vi "StaticTextIndicatorstoSaveSpaceonBlockdiogram_171213.vi"() -> (3 "8":string, 4 "KeyboardShortcuts":string, 5 "KejyboardShortcuts2":string, 6 "Statistics":string, 7 "FilterType":string, 8 "CageSegments":string, 9 "TimeSpentinEachSegment":string, 10 "CageSegmentation":string, 11 "AssignedSegments":string, 12 "Border":string, 13 "Center":string, 14 "CurrentDistanceTraveled":string, 15 "DisplayOptions":string, 16 "3":string, 17 "4":string, 18 "ElapsedTimePlayback":string, 19 "12":string, 20 "13":string, 21 "TIme1":string, 22 "11":string, 23 "Time2":string, 24 "10":string, 25 "ElapsedTimeRecording":string, 26 "5":string)   [LabVIEW 2016]
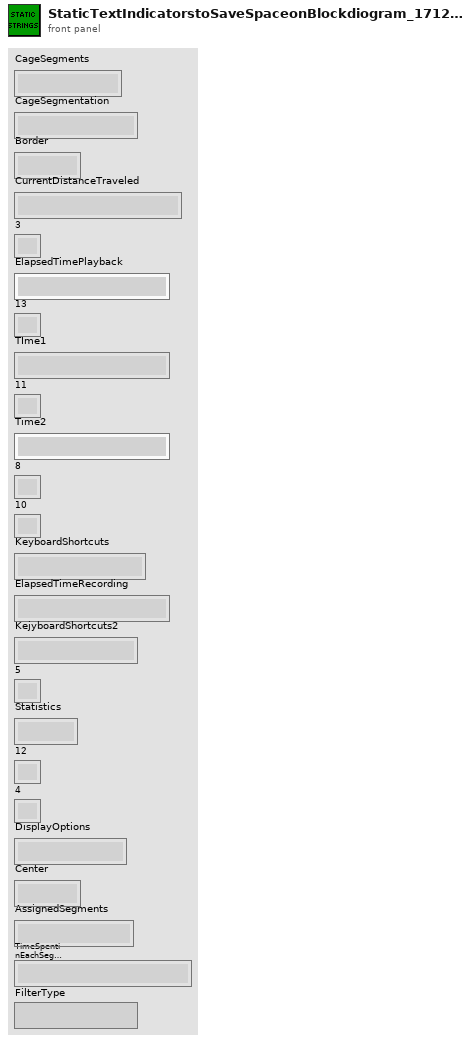
[diagram p1: front panel]
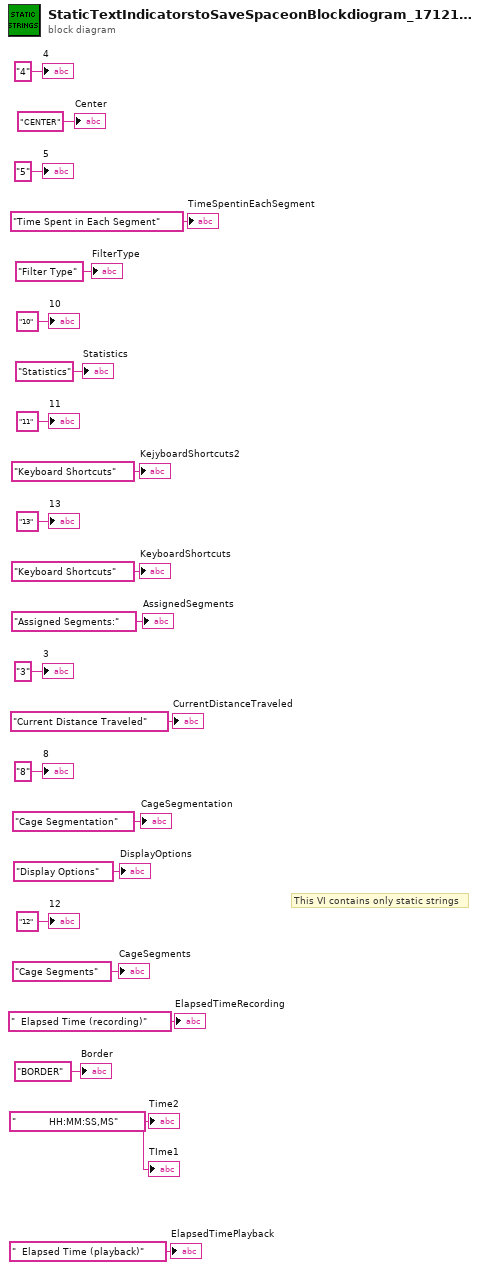
[diagram p0: block diagram]
diagram:
  w6 = "           HH:MM:SS,MS" ("String 5")
  # "This VI contains only static strings"
  "KeyboardShortcuts" <- "Keyboard Shortcuts" ("String 9")
  "Statistics" <- "Statistics" ("String 39")
  "TimeSpentinEachSegment" <- "Time Spent in Each Segment" ("String 40")
  "AssignedSegments" <- "Assigned Segments:" ("String 4")
  "DisplayOptions" <- "Display Options" ("String 35")
  "ElapsedTimeRecording" <- "  Elapsed Time (recording)" ("String")
  "TIme1" <- w6
  "ElapsedTimePlayback" <- "  Elapsed Time (playback)" ("String")
  "Time2" <- w6
  "KejyboardShortcuts2" <- "Keyboard Shortcuts" ("String 30")
  "FilterType" <- "Filter Type" ("String 32")
  "CageSegments" <- "Cage Segments" ("String 8")
  "Border" <- "BORDER" ("String 38")
  "CurrentDistanceTraveled" <- "Current Distance Traveled" ("String 7")
  "8" <- "8" ("String 23")
  "11" <- "11" ("String 26")
  "12" <- "12" ("String 28")
  "Center" <- "CENTER" ("String 36")
  "CageSegmentation" <- "Cage Segmentation" ("String")
  "3" <- "3" ("String 14")
  "4" <- "4" ("String 13")
  "5" <- "5" ("String 12")
  "10" <- "10" ("String 27")
  "13" <- "13" ("String 29")
